vi "GET_WEIGHT.vi"() -> ()   [LabVIEW 2019]
uses:
  <vilib>/Analysis/NI_AALBase.lvlib
panel:
  out "InvalidCommandErr?":bool
  out "variance":dbl format="%0.4f"
  out "standard deviation":dbl format="%0.4f"
  out "mean":dbl format="%0.4f"
  out "tare (g)":dbl[](array[numeric])
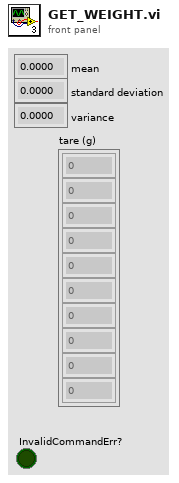
[diagram p1: front panel]
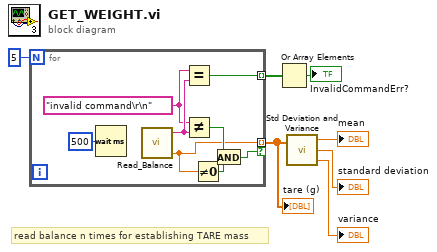
[diagram p0: block diagram]
diagram:
  # "read balance n times for establishing TARE mass"
  n1 = for {
    N: 5 -> [_]
    tunnel: [w8] -> w7 mode=indexing if=w9
    tunnel: [w12] -> w5 mode=indexing
    w13 = "invalid command\r\n"
    n2 = Wait (ms)(milliseconds to wait=u32 500) -> ()  [unwired: 1 out]
    n3 = call "Read_Balance.vi"() -> ("dbl"=w8:dbl, "string"=w14:string)  [unwired: 4 in]
    n4 = Equal?(x=w13, y=w14) -> (x = y?=w12:bool)
    n5 = Not Equal?(x=w13, y=w14) -> (x != y?=w10:bool)
    n6 = Not Equal To 0?(x=w8) -> (x != 0?=w11:bool)
    n7 = And(x=w10, y=w11) -> (x .and. y?=w9:bool)
  }
  "tare (g)" <- w7
  n8 = Or Array Elements(Boolean array=w5) -> (logical OR=→"InvalidCommandErr?":bool)
  n9 = call <vilib>:"Std Deviation and Variance.vi"("X"=w7) -> ("mean"=→"mean":dbl, "standard deviation"=→"standard deviation":dbl, "variance"=→"variance":dbl)  [unwired: 1 in]
